vi "Light.vi"() -> ()   [LabVIEW 2020]
uses:
  <userlib>/_NEVSTOP/Communicable State Machine(CSM)/AdvanceAPI/CSM - Revert Arguments-Safe String.vi
  <userlib>/_NEVSTOP/Communicable State Machine(CSM)/_Shared/Trim Single-line Text.vi
  <userlib>/_NEVSTOP/Communicable State Machine(CSM)/AdvanceAPI/CSM - Make String Arguments Safe.vi
  <userlib>/_NEVSTOP/Communicable State Machine(CSM)/AdvanceAPI/CSM - Break Down Multiple States String.vi
  <userlib>/_NEVSTOP/Communicable State Machine(CSM)/AdvanceAPI/CSM - Compact Multiple States.vi
  <userlib>/_NEVSTOP/Communicable State Machine(CSM)/AdvanceAPI/CSM - Keywords.vi
  <userlib>/_NEVSTOP/Communicable State Machine(CSM)/Communicable State Machine.lvlib
panel:
  out "Boolean":bool
  out "State History":string
  in  "Name (\"\" to Use UUID)":string="Event CSM"
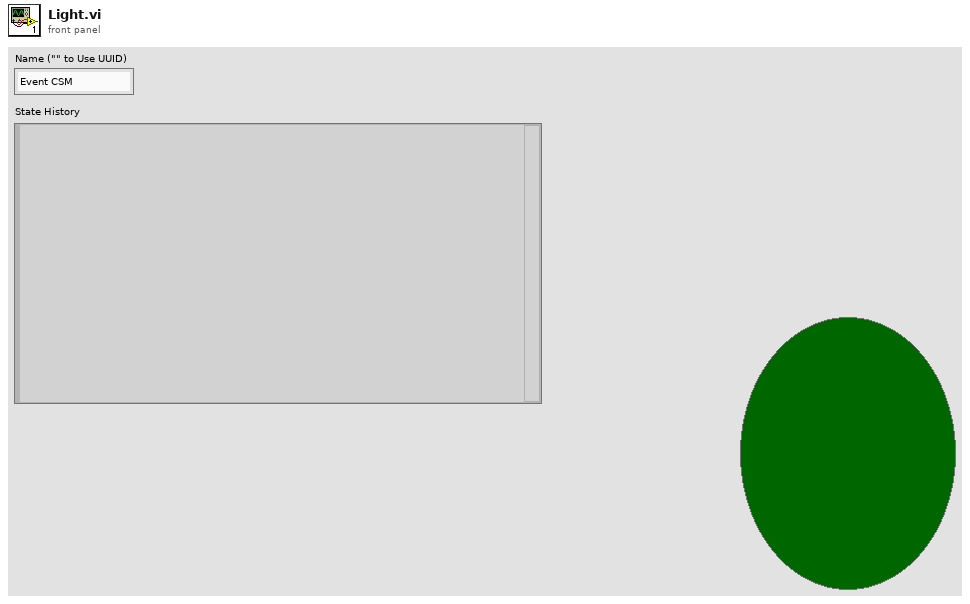
[diagram p1: front panel]
types:
  T1 = enum32{"Invalid", "Standard", "Closed", "Hidden", "Minimized", "Maximized"}
  T2 = enum32{"invalid app kind", "Development System", "Run Time System", "Student Edition", "Embedded LabVIEW", "Evaluation", "Custom"}
  T3 = typedef "Communicable State Machine.lvlib/_CSM_Response Source Message.ctl" = cluster{"‘State":string, "’Arguments":string, "’Error":errorcluster}
  T4 = cluster{"Current VI Reference":refnum<vi>, "Close Panel on Exit?":bool}
  T5 = cluster{"Core":cluster{"Current VI Reference":refnum<vi>, "Close Panel on Exit?":bool}, "Your Boolean data":bool, "Your string data":string}
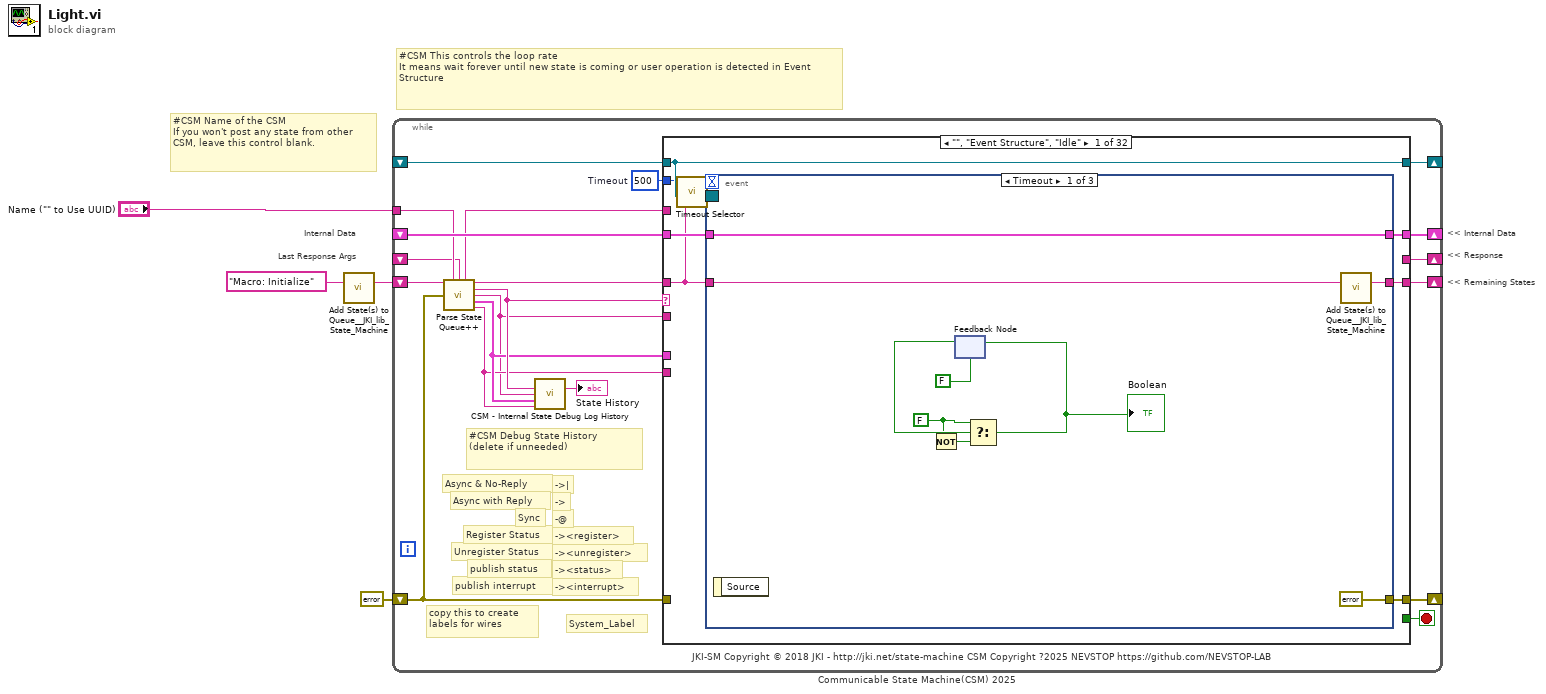
[diagram p0: block diagram]
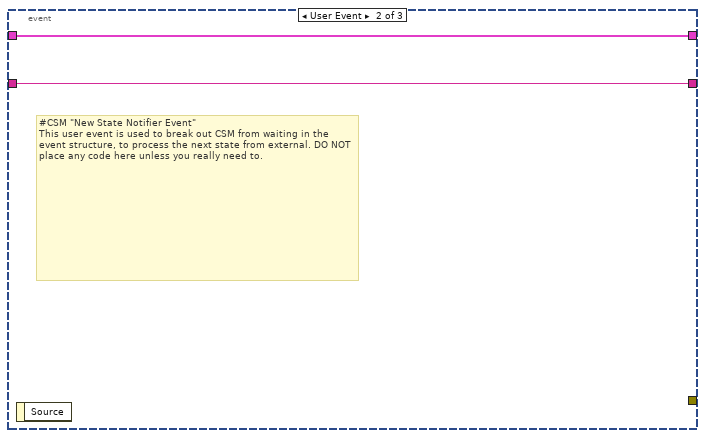
[diagram p2: hidden frame]
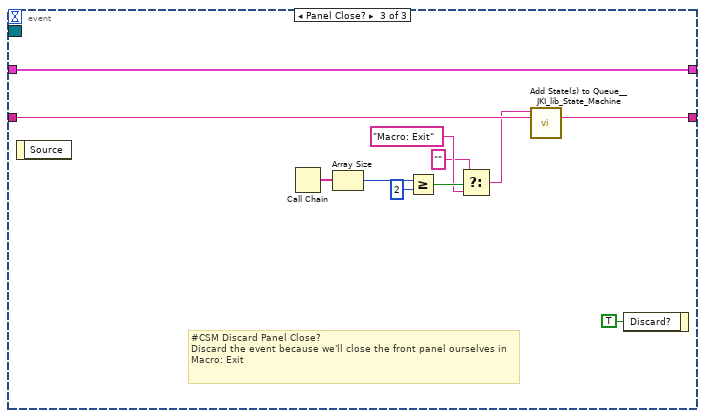
[diagram p3: hidden frame]
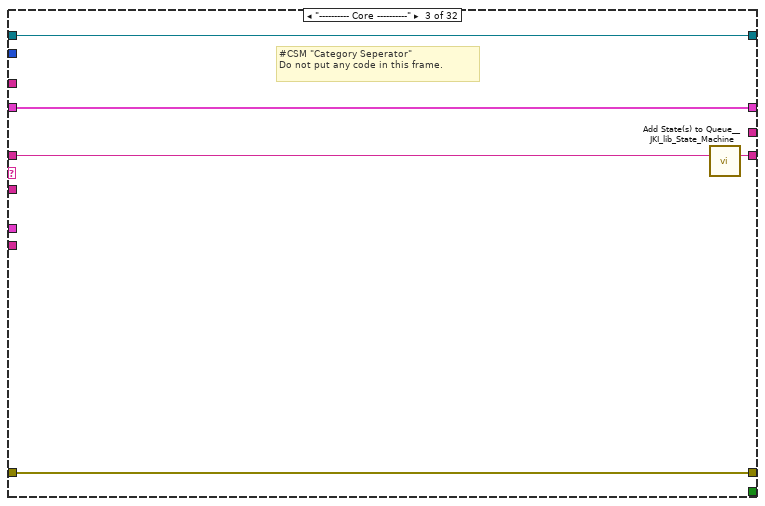
[diagram p5: hidden frame]
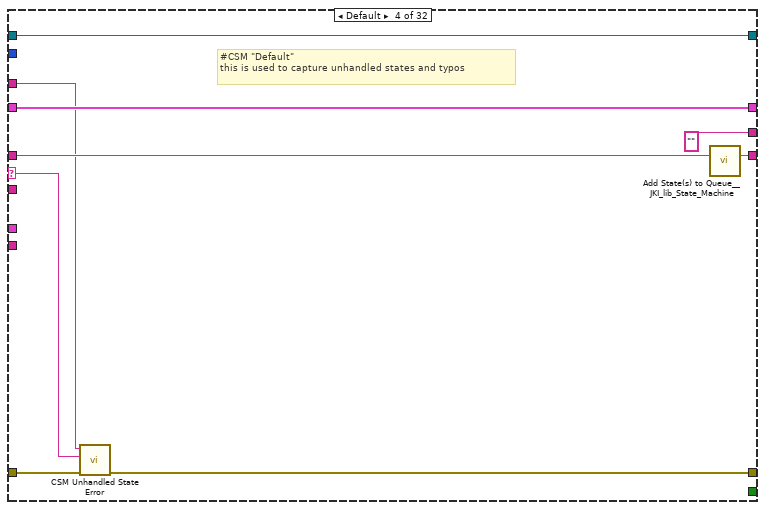
[diagram p6: hidden frame]
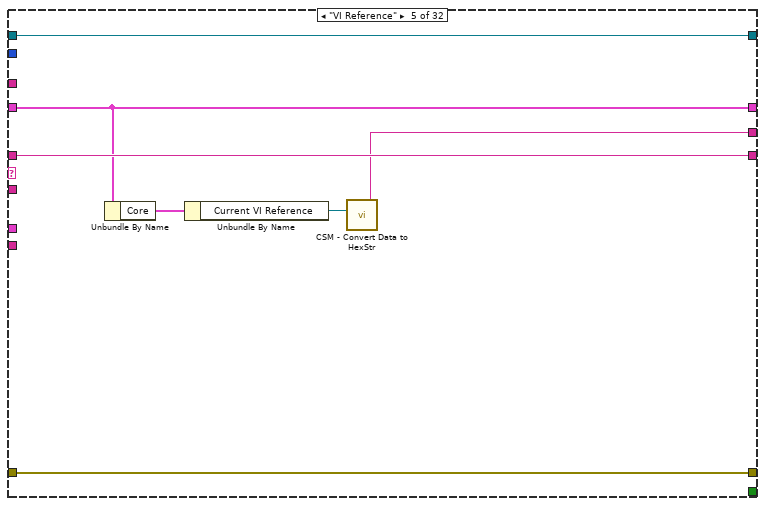
[diagram p7: hidden frame]
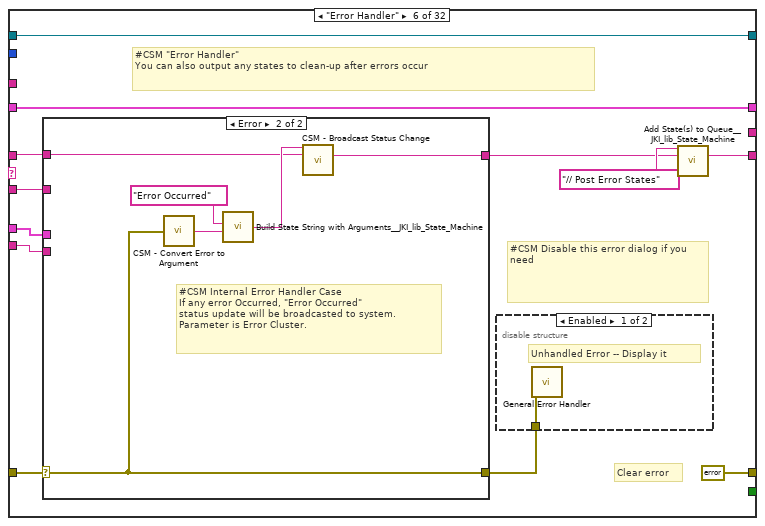
[diagram p8: hidden frame]
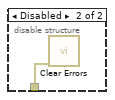
[diagram p9: hidden frame]
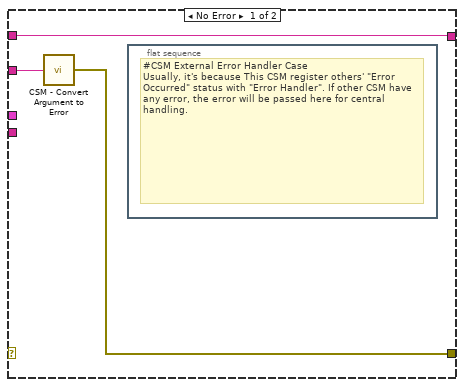
[diagram p10: hidden frame]
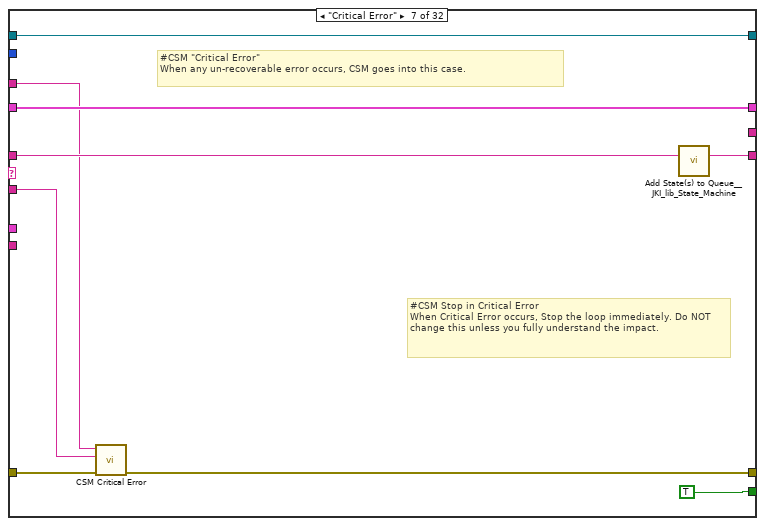
[diagram p11: hidden frame]
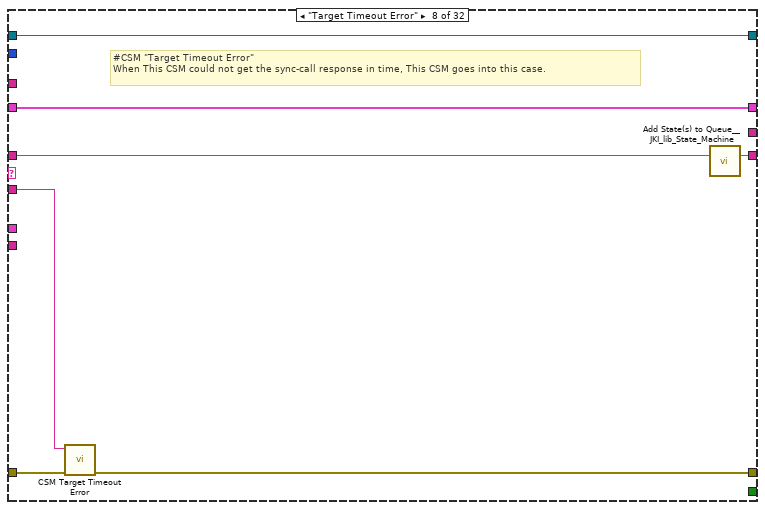
[diagram p12: hidden frame]
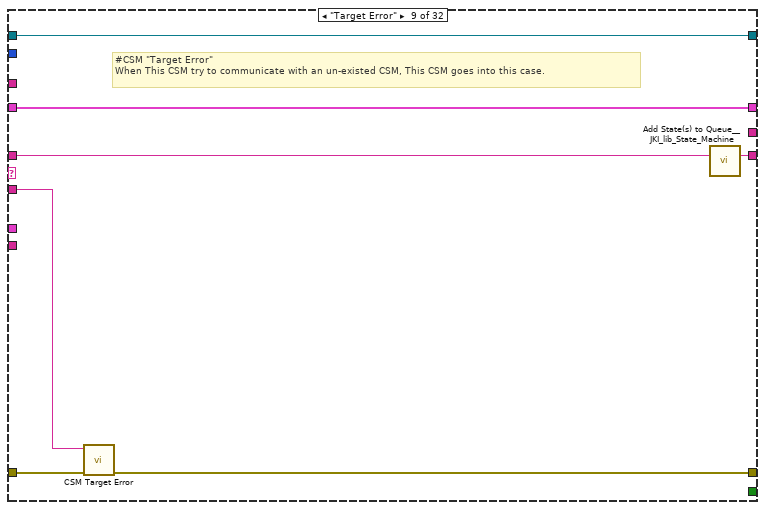
[diagram p13: hidden frame]
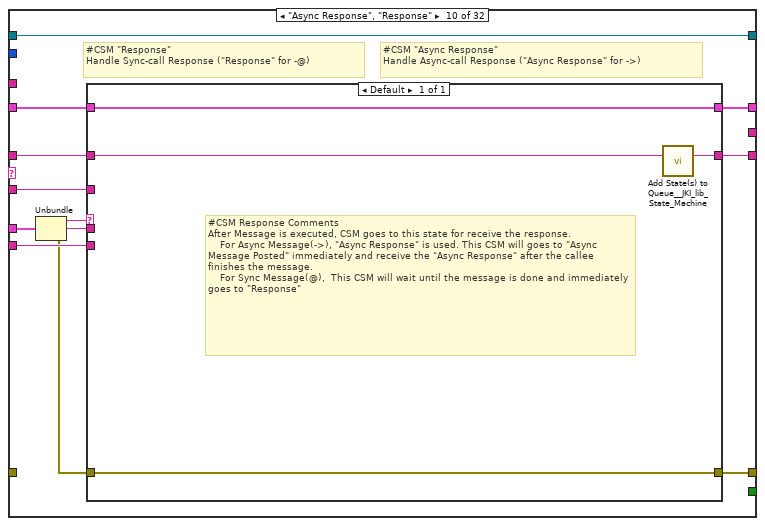
[diagram p14: hidden frame]
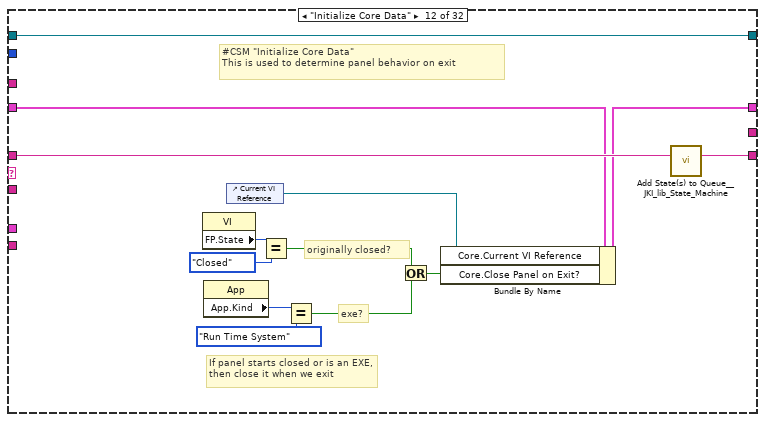
[diagram p16: hidden frame]
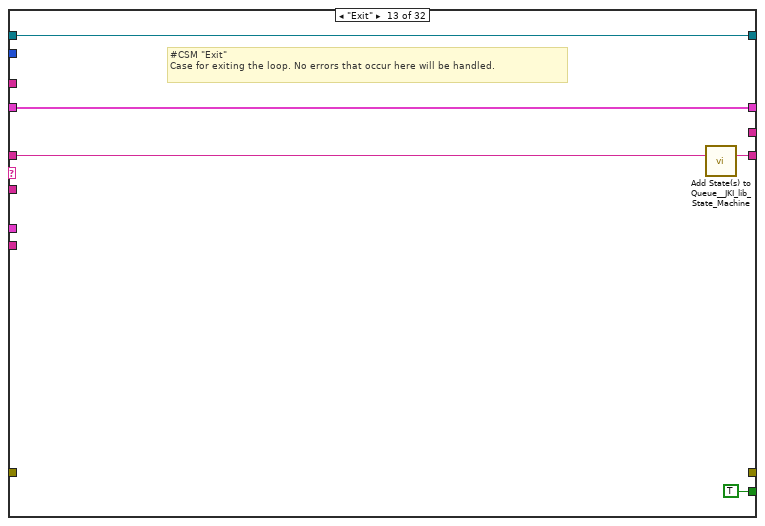
[diagram p17: hidden frame]
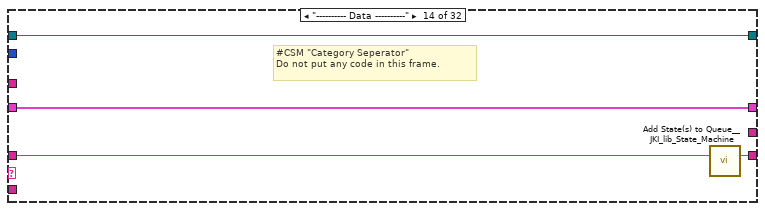
[diagram p18: hidden frame]
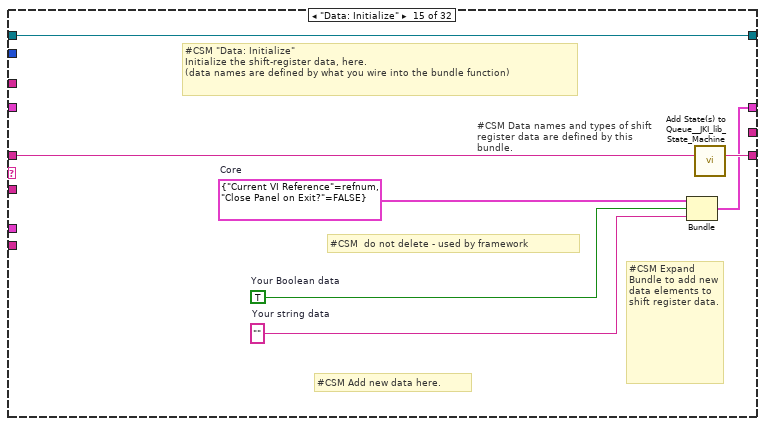
[diagram p19: hidden frame]
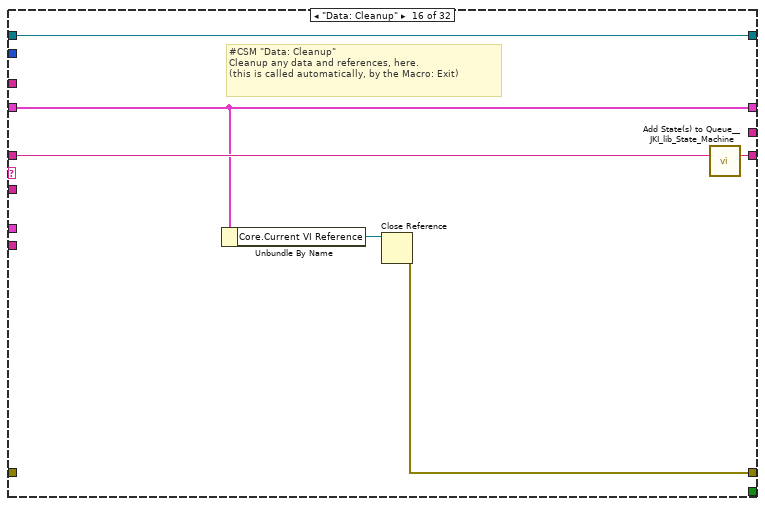
[diagram p20: hidden frame]
diagram:
  # "Last Response Args"
  # "Internal Data"
  # "<< Internal Data"
  # "<< Response"
  # "<< Remaining States"
  # "#CSM Name of the CSM\nIf you won't post any state from other CSM, leave this control blank."
  # "#CSM This controls the loop rate\nIt means wait forever until new state is coming or user operation is detected in Event Structure"
  n1 = call <vilib>:"Add State(s) to Queue__JKI_lib_State_Machine.vi"("State(s) in (\"\")"="Macro: Initialize" ("Init State(\"Macro: Initialize\")")) -> ("States Out"=w1:string)  [unwired: 14 in]
  n2 = while "Communicable State Machine(CSM) 2025" {
    shift-right: [w19] -> _
    shift-left: _ -> [w18]
    shift-right: [w22] -> _
    shift-left: errorcluster {"status"=FALSE, "code"=0, "source"=""} ("error out") -> [w16]
    shift-right: [w21] -> _
    shift-left: w1 -> [w23]
    tunnel: "Name (\"\" to Use UUID)" -> [w12]
    shift-right: [w15] -> _
    shift-left: _ -> [w7]
    shift-right: [w14] -> _
    shift-left: _ -> [w13]
    stop <- w20 stop-if-true
    w17 = 500  # Timeout
    # "#CSM Debug State History\n(delete if unneeded)"
    # "-><interrupt>"
    # "-><status>"
    # "-><unregister>"
    # "-><register>"
    # "-@"
    # "->"
    # "->|"
    # "publish interrupt"
    # "publish status"
    # "Unregister Status"
    # "Register Status"
    # "Sync"
    # "Async with Reply"
    # "Async & No-Reply"
    # "copy this to create labels for wires"
    # "System_Label"
    # "JKI-SM Copyright © 2018 JKI - http://jki.net/state-machine CSM Copyright ?2025 NEVSTOP https://github.com/NEVSTOP-LAB"
    n3 = call <userlib>:"Parse State Queue++.vi"("State Queue"=w23, "Name (\"\" to Use UUID)"=w12, "Response Arguments"=w7, "Previous Error"=w16) -> ("Name Used"=w8:string, "Remaining States"=w24:string, "Current State"=w11:string, "Arguments"=w6:string, "Additional Information"=w10:T3, "Source CSM"=w9:string)  [unwired: 6 in]
    n4 = call <userlib>:"CSM - Internal State Debug Log History.vi"("State"=w11, "Arguments (\"\")"=w6, ">> Response Source Message >>"=w10, "Source (\"\")"=w9) -> ("Debug Log"=→"State History":string)  [unwired: 11 in]
    n5 = case shown="\"\", \"Event Structure\", \"Idle\"" w11 {
      selector: w11 -> [_ _ _ w65 _ _ _ _ _ _ _ _ _ _ _ _ _ _ _ _ _ _ _ _ _ _ _ _ _ _ _ _]
      tunnel: w24 -> [w25 w57 w62 w71 w77 w83 w109 w117 w124 w134 w143 w156 w161 w165 w172 w178 w182 w189 w193 w197 w201 w207 w218 w282 w287 w298 w301 w305 w308 w312 w316 w320]
      tunnel: w6 -> [_ _ _ _ _ w81 w105 w112 w120 w128 _ _ _ _ _ _ _ _ _ _ _ w203 w213 _ _ _ _ _ _ _ _ _]
      tunnel: w18 -> [w31 w56 w59 w69 w76 w89 w110 w115 w122 w132 w142 w150 w159 w163 _ w174 w180 w188 w192 w195 w199 w205 w215 w280 w285 w296 w300 w304 w307 w310 w314 w318]
      tunnel: [w30 _ w60 w63 w78 errorcluster {"status"=FALSE, "code"=0, "source"=""} ("error out") w102 w111 w118 w131 _ _ _ _ _ w175 _ w183 w191 _ _ w204 w216 _ _ _ _ _ _ _ _ _] -> w22
      tunnel: w16 -> [_ _ w60 w64 w78 w87 w103 w113 w119 _ _ _ _ _ _ _ _ _ _ _ _ _ _ _ _ _ _ _ _ _ _ _]
      tunnel: [w32 w57 w61 w70 w77 w85 w108 w116 w123 w135 w143 w155 w160 w164 w171 w177 w181 w189 w193 w196 w200 w206 w217 w281 w286 w297 w301 w305 w308 w311 w315 w319] -> w21
      tunnel: [_ _ _ _ _ _ TRUE _ _ _ _ _ TRUE _ _ _ _ _ _ _ _ _ _ _ _ _ _ _ _ _ _ _] -> w20
      tunnel: [w29 w56 w59 w69 w76 w89 w110 w115 w122 w133 w142 w154 w159 w163 w170 w174 w180 w188 w192 w195 w199 w205 w215 w280 w285 w296 w300 w304 w307 w310 w314 w318] -> w19
      tunnel: w17 -> [w27 _ _ _ _ _ _ _ _ _ _ _ _ _ _ _ _ _ _ _ _ _ _ _ _ _ _ _ _ _ _ _]
      tunnel: w9 -> [_ _ _ _ _ w80 _ _ _ w129 _ _ _ _ _ _ _ _ _ _ _ _ _ _ _ _ _ _ _ _ _ _]
      tunnel: w10 -> [_ _ _ _ _ w79 _ _ _ w130 _ _ _ _ _ _ _ _ _ _ _ _ _ _ _ _ _ _ _ _ _ _]
      tunnel: [_ _ _ "" w72 _ _ _ _ _ _ _ _ _ _ _ _ _ _ _ _ _ _ _ _ _ _ "API1 Response" _ _ _ _] -> w15
      tunnel: [w28 w55 w58 w67 w75 w88 w106 w114 w121 w136 w141 w144 w157 w162 w166 w173 w179 w187 w190 w194 w198 w202 w212 w279 w283 w289 w299 w303 w306 w309 w313 w317] -> w14
      tunnel: w13 -> [w28 w55 w58 w67 w75 w88 w106 w114 w121 w136 w141 w144 w157 w162 w166 w173 w179 _ w190 w194 w198 w202 w212 w279 w283 w289 w299 w303 w306 w309 w313 w317]
      tunnel: w8 -> [_ _ _ w66 _ _ w104 _ _ _ _ _ _ _ _ _ _ w186 _ _ _ _ _ _ _ _ _ _ _ _ _ _]
      frame "", "Event Structure", "Idle" {
        n6 = call <userlib>:"Timeout Selector.vi"("Remaining States"=w25, "Timeout Expected"=w27) -> ("Timeout"=w26:i32)  [unwired: 5 in]
        n7 = event shown="[0] Timeout" {
          selector: w28 -> [_ _ _]
          dyn-events: _ -> [_ _ _]
          timeout: w26 -> [_ _ _]
          tunnel: w25 -> [w41 w42 w54]
          tunnel: [w40 w42 w53] -> w32
          tunnel: w31 -> [w39 w43 w52]
          tunnel: [errorcluster {"status"=FALSE, "code"=0, "source"=""} ("error out") _ _] -> w30
          tunnel: [w39 w43 w52] -> w29
          event Timeout {
            w35 = FALSE
            n8 = event-data() -> ()  [unwired: 1 in, 1 out]
            n9 = Not(x=w35) -> (.not. x?=w34:bool)
            n10 = feedback #1(FALSE) -> (w37:bool)
            n11 = Select(t=w35, s=w37, f=w34) -> (s? t:f=w33:bool)
            "Boolean" <- w33
            n12 = feedback-in #1(w33) -> ()
            n13 = call <vilib>:"Add State(s) to Queue__JKI_lib_State_Machine.vi"("State(s) in (\"\")"=w41) -> ("States Out"=w40:string)  [unwired: 14 in]
          }
          event User Event {
            # "#CSM \"New State Notifier Event\"\nThis user event is used to break out CSM from waiting in the event structure, to process the next state from external. DO NOT place any code here unless you really need to."
            n14 = event-data() -> ()  [unwired: 1 in, 1 out]
          }
          event Panel Close? {
            # "#CSM Discard Panel Close?\nDiscard the event because we'll close the front panel ourselves in Macro: Exit"
            n15 = event-data() -> ()  [unwired: 1 in, 1 out]
            n16 = Call Chain() -> (call chain=w44:string[])
            n17 = Array Size(array=w44) -> (size(s)=w50:i32)
            n18 = Greater Or Equal?(x=w50, y=2) -> (x >= y?=w48:bool)
            n19 = Select(t="", s=w48, f="Macro: Exit") -> (s? t:f=w45:string)
            n20 = call <vilib>:"Add State(s) to Queue__JKI_lib_State_Machine.vi"("State(s) in Front (\"\")"=w45, "State(s) in (\"\")"=w54) -> ("States Out"=w53:string)  [unwired: 13 in]
            n21 = event-data("Discard?"=TRUE) -> ()  [unwired: 1 in, 1 out]
          }
        }
      }
      frame "CSM Documentation" {
        # "#CSM State Syntax\n\n// Comment line, all text to the right of “//” will be ignored\n// Local Message Example\nDoSth: DoA >> Arguments\n\n// Sync Call Example\nAPI: xxxx >> Arguments -@ TargetModule\n\n// Async Call Example\nAPI: xxxx >> Arguments -> TargetModule\n\n// Async Call without Reply Example\nAPI: xxxx >> Arguments ->| TargetModule\n\n// Broadcast normal status:\nStatus >> StatusArguments  -><status>\n\n// Broadcast Interrupt status:\nInterrupt >> StatusArguments  -><interrupt>\n\n// Register Source Module's status to Handler Module\nStatus@Source Module >> Handler Module@Handler Module -><register>\n\n// Unegister Source Module's status\nStatus@Source Module >> Handler Module -><unregister>"
        # "#CSM README FIRST\n\nCommunicable State Machine(CSM) is a LabVIEW application framework that builds upon JKI State Machine(JKISM). It follows the pattern of JKISM and extends the keywords to describe message communication between modules, including concepts such as Sync-Message, Async-Message, Subscription/Unsubscription of status - essential elements for creating reusable code modules. For more information, please visit the CSM wiki: https://nevstop-lab.github.io/CSM-Wiki/\n\nFor instructions on JKI State Machine, visit: \n    http://jki.net/state-machine/\nFor information about CSM, visit: \n    https://github.com/NEVSTOP-LAB"
        # "#CSM \"Documentation\"\nCase for holding CSM Documenation"
      }
      frame "---------- Core ----------" {
        # "#CSM \"Category Seperator\"\nDo not put any code in this frame."
        n22 = call <vilib>:"Add State(s) to Queue__JKI_lib_State_Machine.vi"("State(s) in (\"\")"=w62) -> ("States Out"=w61:string)  [unwired: 14 in]
      }
      frame Default {
        # "#CSM \"Default\"\nthis is used to capture unhandled states and typos"
        n23 = call <userlib>:"CSM Unhandled State Error.vi"("error in (no error)"=w64, "Undefined State"=w65, "CSM Name"=w66) -> ("error out"=w63:errorcluster)  [unwired: 8 in]
        n24 = call <vilib>:"Add State(s) to Queue__JKI_lib_State_Machine.vi"("State(s) in (\"\")"=w71) -> ("States Out"=w70:string)  [unwired: 14 in]
      }
      frame "VI Reference" {
        n25 = Unbundle By Name(w76) -> ("Core"=w74:T4)
        n26 = Unbundle By Name(w74) -> ("Current VI Reference"=w73:refnum<vi>)
        n27 = call <userlib>:"CSM - Convert Data to HexStr.vi"("Variant"=w73) -> ("HEX String (0-9,A-F)"=w72:string)  [unwired: 8 in]
      }
      frame "Error Handler" {
        # "#CSM Disable this error dialog if you need"
        # "#CSM \"Error Handler\"\nYou can also output any states to clean-up after errors occur"
        # "Clear error"
        n28 = case shown="Error" w87 {
          selector: w87 -> [_ w96]
          tunnel: [w94 w98] -> w84
          tunnel: w83 -> [w94 w97]
          tunnel: [w93 w96] -> w82
          tunnel: w81 -> [w95 _]
          tunnel: w80 -> [_ _]
          tunnel: w79 -> [_ _]
          frame No Error {
            n29 = call <userlib>:"CSM - Convert Argument to Error.vi"("Argument"=w95) -> ("Error"=w93:errorcluster)  [unwired: 4 in]
            n30 = flat-sequence {
              frame #0 {
                # "#CSM External Error Handler Case\nUsually, it's because This CSM register others' \"Error Occurred\" status with \"Error Handler\". If other CSM have any error, the error will be passed here for central handling."
              }
            }
          }
          frame Error {
            # "#CSM Internal Error Handler Case \nIf any error Occurred, \"Error Occurred\" \nstatus update will be broadcasted to system.\nParameter is Error Cluster."
            n31 = call <userlib>:"CSM - Convert Error to Argument.vi"("Error"=w96) -> ("Argument"=w100:string)  [unwired: 4 in]
            n32 = call <vilib>:"Build State String with Arguments__JKI_lib_State_Machine.vi"("Arguments (\"\")"=w100, "State"="Error Occurred" ("Status with Arguments")) -> ("State with Arguments"=w99:string)  [unwired: 4 in]
            n33 = call <userlib>:"CSM - Broadcast Status Change.vi"("Status With Arguments"=w99, "State Queue"=w97) -> ("Remaining States"=w98:string)  [unwired: 13 in]
          }
        }
        n34 = disable-structure shown="Enabled" {
          disable-tunnel: w82 -> [w91 w92]
          frame Enabled {
            # "Unhandled Error -- Display it"
            n35 = call <vilib>:"General Error Handler.vi"("error in (no error)"=w91) -> ()  [unwired: 10 in, 5 out]
          }
          frame Disabled {
            n36 = call <vilib>:"Clear Errors.vi"("error in (no error)"=w92) -> ()  [unwired: 5 in, 2 out]
          }
        }
        n37 = call <vilib>:"Add State(s) to Queue__JKI_lib_State_Machine.vi"("State(s) in Front (\"\")"="// Post Error States", "State(s) in (\"\")"=w84) -> ("States Out"=w85:string)  [unwired: 13 in]
      }
      frame "Critical Error" {
        # "#CSM \"Critical Error\"\nWhen any un-recoverable error occurs, CSM goes into this case."
        # "#CSM Stop in Critical Error\nWhen Critical Error occurs, Stop the loop immediately. Do NOT change this unless you fully understand the impact."
        n38 = call <userlib>:"CSM Critical Error.vi"("error in (no error)"=w103, "Arugments (As Reason)"=w105, "CSM Name"=w104) -> ("error out"=w102:errorcluster)  [unwired: 8 in]
        n39 = call <vilib>:"Add State(s) to Queue__JKI_lib_State_Machine.vi"("State(s) in (\"\")"=w109) -> ("States Out"=w108:string)  [unwired: 14 in]
      }
      frame "Target Timeout Error" {
        # "#CSM \"Target Timeout Error\"\nWhen This CSM could not get the sync-call response in time, This CSM goes into this case."
        n40 = call <userlib>:"CSM Target Timeout Error.vi"("error in (no error)"=w113, "Arguments (As CSM Name)"=w112) -> ("error out"=w111:errorcluster)  [unwired: 9 in]
        n41 = call <vilib>:"Add State(s) to Queue__JKI_lib_State_Machine.vi"("State(s) in (\"\")"=w117) -> ("States Out"=w116:string)  [unwired: 14 in]
      }
      frame "Target Error" {
        # "#CSM \"Target Error\"\nWhen This CSM try to communicate with an un-existed CSM, This CSM goes into this case."
        n42 = call <userlib>:"CSM Target Error.vi"("error in (no error)"=w119, "Arguments (As CSM Name)"=w120) -> ("error out"=w118:errorcluster)  [unwired: 9 in]
        n43 = call <vilib>:"Add State(s) to Queue__JKI_lib_State_Machine.vi"("State(s) in (\"\")"=w124) -> ("States Out"=w123:string)  [unwired: 14 in]
      }
      frame "Async Response", "Response" {
        # "#CSM \"Async Response\"\nHandle Async-call Response (\"Async Response\" for ->)"
        # "#CSM \"Response\"\nHandle Sync-call Response (\"Response\" for -@)"
        n44 = Unbundle(w130) -> ("‘State"=w127:string, "’Arguments"=w126:string, "’Error"=w125:errorcluster)
        n45 = case shown="Default" w127 {
          tunnel: [w137] -> w135
          tunnel: w134 -> [w138]
          tunnel: [w140] -> w133
          tunnel: w132 -> [w140]
          tunnel: [w139] -> w131
          tunnel: w125 -> [w139]
          tunnel: w129 -> [_]
          tunnel: w128 -> [_]
          tunnel: w126 -> [_]
          frame Default {
            # "#CSM Response Comments\nAfter Message is executed, CSM goes to this state for receive the response.\n    For Async Message(->), \"Async Response\" is used. This CSM will goes to \"Async Message Posted\" immediately and receive the \"Async Response\" after the callee finishes the message.\n    For Sync Message(@),  This CSM will wait until the message is done and immediately goes to \"Response\""
            n46 = call <vilib>:"Add State(s) to Queue__JKI_lib_State_Machine.vi"("State(s) in (\"\")"=w138) -> ("States Out"=w137:string)  [unwired: 14 in]
          }
        }
      }
      frame "Async Message Posted" {
        # "#CSM \"Async Message Posted\"\nAfter Async Message is posted (-> or ->| ), CSM goes to this state for post-action.\nYou can use Argument - State to tell which Async Message is called."
      }
      frame "Initialize Core Data" {
        # "#CSM \"Initialize Core Data\"\nThis is used to determine panel behavior on exit"
        # "originally closed?"
        # "exe?"
        # "If panel starts closed or is an EXE, then close it when we exit"
        n47 = property class="VI"() -> ("FP.State"=w147:T1)  [unwired: 2 in, 2 out]
        n48 = property class="App"() -> ("App.Kind"=w153:T2)  [unwired: 2 in, 2 out]
        n49 = control-ref of="Current VI Reference"() -> (w148:refnum<vi>)
        n50 = Equal?(x=w147, y=T1."Closed" ("Front Panel Window:State")) -> (x = y?=w145:bool)
        n51 = Equal?(x=w153, y=T2."Run Time System" ("Application:Kind")) -> (x = y?=w151:bool)
        n52 = Or(x=w145, y=w151) -> (x .or. y?=w149:bool)
        n53 = Bundle By Name(cluster=w150, "Core.Current VI Reference"=w148, "Core.Close Panel on Exit?"=w149) -> (w154:T5)
        n54 = call <vilib>:"Add State(s) to Queue__JKI_lib_State_Machine.vi"("State(s) in (\"\")"=w156) -> ("States Out"=w155:string)  [unwired: 14 in]
      }
      frame "Exit" {
        # "#CSM \"Exit\"\nCase for exiting the loop. No errors that occur here will be handled."
        n55 = call <vilib>:"Add State(s) to Queue__JKI_lib_State_Machine.vi"("State(s) in (\"\")"=w161) -> ("States Out"=w160:string)  [unwired: 14 in]
      }
      frame "---------- Data ----------" {
        # "#CSM \"Category Seperator\"\nDo not put any code in this frame."
        n56 = call <vilib>:"Add State(s) to Queue__JKI_lib_State_Machine.vi"("State(s) in (\"\")"=w165) -> ("States Out"=w164:string)  [unwired: 14 in]
      }
      frame "Data: Initialize" {
        w167 = T4 {"Current VI Reference"=refnum, "Close Panel on Exit?"=FALSE}  # Core
        w169 = TRUE  # Your Boolean data
        w168 = ""  # Your string data
        # "#CSM  do not delete - used by framework"
        # "#CSM Expand Bundle to add new data elements to shift register data."
        # "#CSM Add new data here."
        # "#CSM Data names and types of shift register data are defined by this bundle."
        # "#CSM \"Data: Initialize\"\nInitialize the shift-register data, here.\n(data names are defined by what you wire into the bundle function)"
        n57 = Bundle("Core"=w167, "Your Boolean data"=w169, "Your string data"=w168) -> (w170:T5)  [unwired: 1 in]
        n58 = call <vilib>:"Add State(s) to Queue__JKI_lib_State_Machine.vi"("State(s) in (\"\")"=w172) -> ("States Out"=w171:string)  [unwired: 14 in]
      }
      frame "Data: Cleanup" {
        # "#CSM \"Data: Cleanup\"\nCleanup any data and references, here.\n(this is called automatically, by the Macro: Exit)"
        n59 = Unbundle By Name(w174) -> ("Core.Current VI Reference"=w176:refnum<vi>)
        n60 = Close Reference(reference=w176) -> (error out=w175:errorcluster)  [unwired: 1 in]
        n61 = call <vilib>:"Add State(s) to Queue__JKI_lib_State_Machine.vi"("State(s) in (\"\")"=w178) -> ("States Out"=w177:string)  [unwired: 14 in]
      }
      frame "---------- Events ----------" {
        # "#CSM \"Category Seperator\"\nDo not put any code in this frame."
        n62 = call <vilib>:"Add State(s) to Queue__JKI_lib_State_Machine.vi"("State(s) in (\"\")"=w182) -> ("States Out"=w181:string)  [unwired: 14 in]
      }
      frame "Events: Register" {
        # "#CSM \"Events: Register\"\nRegister user event. New Message Event is registered to break CSM waiting in event structure by default."
        # "#CSM Register New Message Event\nRegister message event to break Waiting in Event structure."
        n63 = call <userlib>:"CSM - Get New State Notifier Event.vi"("Name (\"\" to Use UUID)"=w186) -> ("error out"=w184:errorcluster, "New State Notifier Event"=w185:refnum<user-event>)  [unwired: 9 in]
        n64 = register-events(error in=w184, w185) -> (reference out=w187:refnum<event-registration>, error out=w183:errorcluster)  [unwired: 1 in]
      }
      frame "Events: Unregister" {
        # "#CSM \"Events: Unregister\"\nUnregister user event."
        n65 = Unregister For Events(event registration refnum=w190) -> (error out=w191:errorcluster)  [unwired: 1 in]
      }
      frame "---------- UI ----------" {
        # "#CSM \"Category Seperator\"\nDo not put any code in this frame."
        n66 = call <vilib>:"Add State(s) to Queue__JKI_lib_State_Machine.vi"("State(s) in (\"\")"=w197) -> ("States Out"=w196:string)  [unwired: 14 in]
      }
      frame "UI: Initialize" {
        # "#CSM \"UI: Initialize\"\nInitialize the User Interface, here.\n(this is called automatically, by the Macro: Init)"
        n67 = call <vilib>:"Add State(s) to Queue__JKI_lib_State_Machine.vi"("State(s) in (\"\")"=w201) -> ("States Out"=w200:string)  [unwired: 14 in]
      }
      frame "UI: Cursor Set" {
        # "Argument"
        # "#CSM \"UI: Cursor Set\"\nSet and Unset Cursor Busy.\n(Usage: \"UI: Cursor Set >> Busy|Idle\")"
        n68 = disable-structure shown="TARGET_TYPE!=Windows" {
          disable-tunnel: [w209 _] -> w204
          disable-tunnel: w203 -> [w208 _]
          frame condition #0 (active) {
            n69 = case shown="\"Idle\", Default" w208 {
              tunnel: [w210 w211] -> w209
              frame "Idle", Default {
                n70 = call <vilib>:"Unset Busy.vi"() -> ("error out"=w210:errorcluster)  [unwired: 11 in]
              }
              frame "Busy" {
                n71 = call <vilib>:"Set Busy.vi"() -> ("error out"=w211:errorcluster)  [unwired: 10 in, 1 out]
              }
            }
          }
          frame condition #1 {
          }
        }
        n72 = call <vilib>:"Add State(s) to Queue__JKI_lib_State_Machine.vi"("State(s) in (\"\")"=w207) -> ("States Out"=w206:string)  [unwired: 14 in]
      }
      frame "UI: Front Panel State" {
        # "Argument"
        # "#CSM \"UI: Front Panel State\"\nSet Front Panel Open or Closed\n(Usage: \"UI: Front Panel State >> Open|Close\")"
        n73 = Unbundle By Name(w215) -> ("Core.Current VI Reference"=w214:refnum<vi>)
        n74 = case shown="\"Open\", \"Standard\", Default" w213 {
          tunnel: [w225 w238 w249 w261 w273] -> w216
          tunnel: w214 -> [w224 w236 w248 w260 w272]
          frame "Open", "Standard", Default {
            w219 = T1."Standard" ("State")
            n75 = property class="VI"(reference=w224) -> (reference out=w222:refnum<vi>, error out=w223:errorcluster, "FP.State"=w221:T1)  [unwired: 1 in]
            n76 = Not Equal?(x=w221, y=w219) -> (x != y?=w220:bool)
            n77 = case shown="True" w220 {
              tunnel: [w229 w231] -> w225
              tunnel: w223 -> [w228 w231]
              tunnel: w222 -> [w227 _]
              tunnel: w219 -> [w226 _]
              frame True {
                n78 = invoke class="VI" method="FP.Open"(reference=w227, error in=w228, "Activate"=TRUE, "State"=w226) -> (error out=w229:errorcluster)  [unwired: 1 in, 4 out]
              }
              frame False {
              }
            }
          }
          frame "Close", "Closed" {
            n79 = property class="VI"(reference=w236) -> (reference out=w235:refnum<vi>, error out=w237:errorcluster, "FP.State"=w233:T1)  [unwired: 1 in]
            n80 = Not Equal?(x=w233, y=T1."Closed" ("Front Panel Window:State")) -> (x != y?=w232:bool)
            n81 = case shown="True" w232 {
              tunnel: [w239 w242] -> w238
              tunnel: w237 -> [w239 w241]
              tunnel: w235 -> [_ w240]
              frame False {
              }
              frame True {
                n82 = invoke class="VI" method="FP.Close"(reference=w240, error in=w241) -> (error out=w242:errorcluster)  [unwired: 1 in, 2 out]
              }
            }
          }
          frame "Hidden", "Hide" {
            w243 = T1."Hidden" ("State")
            n83 = property class="VI"(reference=w248) -> (reference out=w246:refnum<vi>, error out=w247:errorcluster, "FP.State"=w245:T1)  [unwired: 1 in]
            n84 = Not Equal?(x=w245, y=w243) -> (x != y?=w244:bool)
            n85 = case shown="True" w244 {
              tunnel: [w253 w254] -> w249
              tunnel: w247 -> [w252 w254]
              tunnel: w246 -> [w251 _]
              tunnel: w243 -> [w250 _]
              frame True {
                n86 = invoke class="VI" method="FP.Open"(reference=w251, error in=w252, "State"=w250) -> (error out=w253:errorcluster)  [unwired: 2 in, 4 out]
              }
              frame False {
              }
            }
          }
          frame "Minimize", "Minimized" {
            w255 = T1."Minimized" ("State")
            n87 = property class="VI"(reference=w260) -> (reference out=w258:refnum<vi>, error out=w259:errorcluster, "FP.State"=w257:T1)  [unwired: 1 in]
            n88 = Not Equal?(x=w257, y=w255) -> (x != y?=w256:bool)
            n89 = case shown="False" w256 {
              tunnel: [w265 w266] -> w261
              tunnel: w259 -> [w264 w266]
              tunnel: w258 -> [w263 _]
              tunnel: w255 -> [w262 _]
              frame True {
                n90 = invoke class="VI" method="FP.Open"(reference=w263, error in=w264, "State"=w262) -> (error out=w265:errorcluster)  [unwired: 2 in, 4 out]
              }
              frame False {
              }
            }
          }
          frame "Maximize", "Maximized" {
            w267 = T1."Maximized" ("State")
            n91 = property class="VI"(reference=w272) -> (reference out=w270:refnum<vi>, error out=w271:errorcluster, "FP.State"=w269:T1)  [unwired: 1 in]
            n92 = Not Equal?(x=w269, y=w267) -> (x != y?=w268:bool)
            n93 = case shown="True" w268 {
              tunnel: [w277 w278] -> w273
              tunnel: w271 -> [w276 w278]
              tunnel: w270 -> [w275 _]
              tunnel: w267 -> [w274 _]
              frame True {
                n94 = invoke class="VI" method="FP.Open"(reference=w275, error in=w276, "State"=w274) -> (error out=w277:errorcluster)  [unwired: 2 in, 4 out]
              }
              frame False {
              }
            }
          }
        }
        n95 = call <vilib>:"Add State(s) to Queue__JKI_lib_State_Machine.vi"("State(s) in (\"\")"=w218) -> ("States Out"=w217:string)  [unwired: 14 in]
      }
      frame "---------- Macro ----------" {
        # "#CSM \"Category Seperator\"\nDo not put any code in this frame."
        n96 = call <vilib>:"Add State(s) to Queue__JKI_lib_State_Machine.vi"("State(s) in (\"\")"=w282) -> ("States Out"=w281:string)  [unwired: 14 in]
      }
      frame "Macro: Initialize" {
        w284 = "Data: Initialize\nInitialize Core Data\nEvents: Register\nUI: Initialize\n//UI: Front Panel State >> Open"  # Data: Initialize Initialize Core Data Events: Register UI: Initialize //UI: Front Panel State >> Open
        # "#CSM \"Macro: Initialize\"\nInitialization Macro (This is called once, when the VI starts)"
        n97 = call <vilib>:"Add State(s) to Queue__JKI_lib_State_Machine.vi"("State(s) in Front (\"\")"=w284, "State(s) in (\"\")"=w287) -> ("States Out"=w286:string)  [unwired: 13 in]
      }
      frame "Macro: Exit" {
        # "#CSM \"Macro: Exit\"\nExit Macro (This is called once, when the VI exits)"
        n98 = Unbundle By Name(w296) -> ("Core.Close Panel on Exit?"=w295:bool)
        n99 = Select(t="UI: Front Panel State >> Close", s=w295, f="") -> (s? t:f=w292:string)
        n100 = call <vilib>:"Add State(s) to Queue__JKI_lib_State_Machine.vi"("State(s) in Front (\"\")"="//Exit Sub-Modules ", "State(s) in (\"\")"=w292, "State(s) at Back (\"\")"="Data: Cleanup\nEvents: Unregister\nExit") -> ("States Out"=w290:string)  [unwired: 12 in]
        n101 = call <vilib>:"Add State(s) to Queue__JKI_lib_State_Machine.vi"("State(s) in Front (\"\")"=w290, "State(s) in (\"\")"=w298) -> ("States Out"=w297:string)  [unwired: 13 in]
      }
      frame "---------- API ----------" {
        # "#CSM \"Category Seperator\"\nDo not put any code in this frame."
      }
      frame "API: API1" {
        # "#CSM >> Source CSM >>\nIf you need to tell who triggered this state , use this string. If it's this case itself, this string is \"\"."
        # "#CSM >> Arguments >>\nDeal with the parameter if any"
        # "#CSM Response\nConnect this to return the response of your API"
        # "#CSM API Example\nCopy/Rename this case for your own API"
      }
      frame "API: API2" {
        # "#CSM API Example\nCopy/Rename this case for your own API"
      }
      frame "---------- Action ----------" {
        # "#CSM \"Category Seperator\"\nDo not put any code in this frame."
        n102 = call <vilib>:"Add State(s) to Queue__JKI_lib_State_Machine.vi"("State(s) in (\"\")"=w312) -> ("States Out"=w311:string)  [unwired: 14 in]
      }
      frame "Action: action1" {
        # "#CSM \"Internal State\"\nThis category is used for holding internal states"
        n103 = call <vilib>:"Add State(s) to Queue__JKI_lib_State_Machine.vi"("State(s) in (\"\")"=w316) -> ("States Out"=w315:string)  [unwired: 14 in]
      }
      frame "Action: action2" {
        # "#CSM \"Internal State\"\nThis category is used for holding internal states"
        n104 = call <vilib>:"Add State(s) to Queue__JKI_lib_State_Machine.vi"("State(s) in (\"\")"=w320) -> ("States Out"=w319:string)  [unwired: 14 in]
      }
    }
  }
